vi "Load_Destination_Type.vi"(8 "error in (no error)":errorcluster, 9 "index":i32, 11 "buildObject":T1) -> (0 "error out":errorcluster, 3 "AB_Destination out":refnum<class "AB_Destination.lvclass">)   [LabVIEW 2020, in "AB_Destination.lvclass"]
uses:
  <vilib>/AppBuilder/AB_Classes/Destination/AB_Destination.lvclass
  <resource>/Framework/Providers/API/ItemRef.ctl
  <vilib>/AppBuilder/AB_Classes/Destination/Dest_LLB/AB_Dest_LLB.lvclass
  e:/builds/penguin/labview/branches/2020/dev/dist/vi.lib/AppBuilder/AB_Classes/Destination/AB_Destination.lvclass
  <vilib>/AppBuilder/AB_Classes/Destination/Dest_Application/AB_Dest_App.lvclass
  <vilib>/AppBuilder/AB_Classes/Destination/Dest_LegacyApplication/AB_Dest_LegacyApp.lvclass
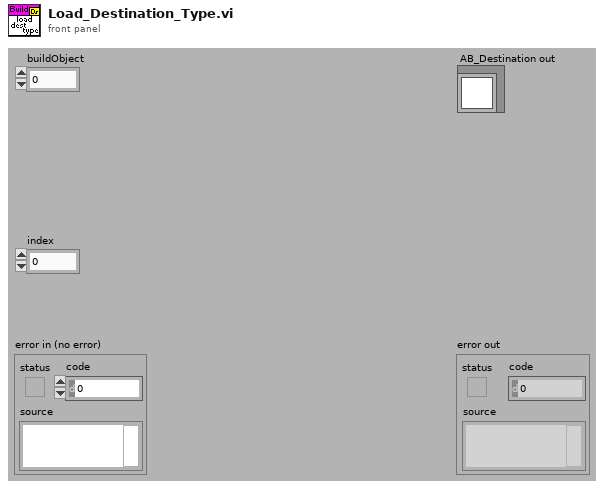
[diagram p1: front panel]
types:
  T1 = typedef "ItemRef.ctl" = u64
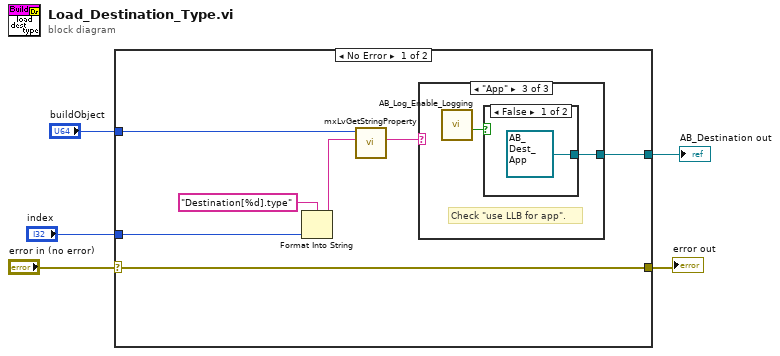
[diagram p0: block diagram]
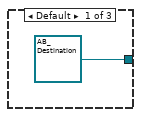
[diagram p2: hidden frame]
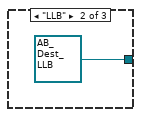
[diagram p3: hidden frame]
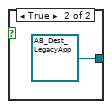
[diagram p4: hidden frame]
diagram:
  n1 = case shown="No Error" "error in (no error)" {
    selector: "error in (no error)" -> [w12 w19]
    tunnel: [w12 w19] -> w4
    tunnel: [w6 _] -> w3
    tunnel: "buildObject" -> [w10 _]
    tunnel: "index" -> [w9 _]
    frame No Error {
      n2 = Format Into String(format string="Destination[%d].type", w9) -> (resulting string=w8:string)  [unwired: 2 in, 1 out]
      n3 = call <resource>:"mxLvGetStringProperty.vi"("Tag"=w8, "Item"=w10) -> ("Value"=w7:string)  [unwired: 1 in, 8 out]
      n4 = case shown="\"App\"" w7 {
        tunnel: [refnum<class "AB_Destination.lvclass"> refnum ("AB_Destination in") refnum<class "AB_Dest_LLB.lvclass"> refnum ("AB_Dest_LLB.lvclass") w15] -> w6
        frame Default {
        }
        frame "LLB" {
        }
        frame "App" {
          # "Check \"use LLB for app\"."
          n5 = call <vilib>:"AB_Log_Enable_Logging.vi"() -> ("use LLB for app"=w16:bool)  [unwired: 2 in, 9 out]
          n6 = case shown="False" w16 {
            tunnel: [refnum<class "AB_Dest_App.lvclass"> refnum ("AB_Dest_App.lvclass") refnum<class "AB_Dest_LegacyApp.lvclass"> refnum ("AB_Dest_LegacyApp.lvclass")] -> w15
            frame False {
            }
            frame True {
            }
          }
        }
      }
    }
    frame Error {
    }
  }
  "error out" <- w4
  "AB_Destination out" <- w3
